vi "peg in hole Summary.vi"() -> ()   [LabVIEW 2013]
uses:
  <vilib>/Utility/file.llb/Write To Spreadsheet File (string).vi
  <vilib>/Utility/file.llb/Write To Spreadsheet File (DBL).vi
panel:
  in  "2015-03-02":dbl[](array[numeric])=[27.75, 28.05, 27.9, 17.75, 143.25, 110.6, 42.95, 17.2, 41.6, 16.8, 27.95, 65.9, 30.25, 18.5, 17.5, 48.1, 62.35, 17.55, 52.75, 322.0, 27.9, 27.45, 27.2, 18.0, 17.4, 27.95, 51.2, 17.55, 40.2, 171.4, 28.25, 27.85, 27.35, 17.85, 16.95, 39.3, 38.75, 17.35, 29.45, 17.2, 27.8, 28.15, 142.2, 63.6, 17.65, 89.651, 28.5, 17.55, 29.0, 17.15, 17.65, 28.45, 28.45, 42.9, 16.75, 38.55, 39.45, 17.8, 208.85, 49.9, 17.25, 37.75, 69.85, 29.9, 17.3, 17.5, 19.1, 80.35, 31.499, 80.55, 17.45, 17.65, 27.95, 40.65, 17.25, 70.15, 28.8, 17.4, 18.4, 17.55, 16.95, 50.4, 27.15, 52.5, 16.85, 17.6, 39.6, 17.35, 18.35, 17.75, 58.15, 71.55, 27.65, 107.75, 16.95, 28.75, 28.7, 17.5, 128.9, 59.35]
  in  "1 taught Point":dbl[](array[numeric])=[35.801, 15.05, 145.25, 25.05, 85.2, 31.05, 196.6, 25.1, 135.5, 25.45, 125.65, 25.3, 55.75, 147.2, 64.85, 25.35, 116.2, 35.45, 85.7, 45.3, 35.3, 15.9, 35.25, 15.45, 65.45, 15.35, 55.35, 14.55, 339.85, 14.65, 86.2, 15.7, 45.45, 15.449, 74.949, 26.0, 68.55, 36.45, 36.2, 26.55, 57.05, 16.65, 25.649, 58.1, 111.0, 25.9, 15.3, 129.8, 55.5, 15.3, 35.3, 15.25, 14.85, 14.55, 35.3, 15.35, 14.95, 15.25, 25.15, 14.6, 14.65, 25.6, 38.05, 15.95, 35.25, 14.75, 35.1, 15.15, 36.05, 15.1, 35.55, 14.85, 25.65, 36.9, 15.1, 14.9, 85.45, 14.5, 37.3, 14.6, 15.3, 15.35, 45.35, 15.25, 65.75, 35.85, 25.25, 15.6, 25.15, 15.35, 15.15, 36.3, 55.95, 15.5, 25.1, 14.5, 96.5, 14.8, 35.2, 14.5, 15.35, 15.65, 15.0, 15.25, 66.8, 15.4, 15.0, 15.35, 15.0, 15.35, 15.3, 15.4, 15.15, 15.35, 14.9, 15.2, 15.05, 15.4, 25.05, 14.65, 14.9, 15.45, 15.2, 15.35, 15.05, 15.45, 55.7, 15.15, 15.05, 15.5, 15.25, 15.65, 46.1, 15.6, 15.0, 15.05, 14.9, 15.4, 14.95, 15.0]
  in  "2 taught points":dbl[](array[numeric])=[126.95, 36.6, 65.75, 57.35, 75.85, 36.85, 25.5, 26.1, 45.8, 158.25, 25.35, 15.7, 127.05, 98.35, 76.5, 46.15, 85.8, 57.7, 54.95, 47.9, 35.75, 47.35, 66.2, 15.35, 116.3, 26.45, 66.45, 16.0, 55.95, 26.9, 148.35, 47.152, 140.1, 16.201, 65.8, 15.45, 45.25, 36.95, 35.7, 15.75, 57.499, 15.75, 36.25, 122.1, 68.25, 203.25, 36.0, 68.1, 75.65, 88.2, 75.45, 99.4, 55.4, 108.6, 45.65, 99.1, 35.75, 173.4, 35.6, 89.5, 45.9, 183.05, 35.6, 110.95, 35.4, 129.85, 35.6, 67.4, 36.15, 77.05, 35.35, 171.55, 25.2, 78.45, 98.95, 15.2, 25.05, 170.75, 35.65, 67.3, 77.85, 66.65, 65.85, 130.9, 25.1, 110.35, 46.051, 15.15, 66.35, 297.45, 25.15, 150.4, 88.0, 113.1, 36.5, 90.75, 25.75, 143.35, 56.5, 78.4, 47.55, 310.05, 15.052, 77.5, 27.3, 67.6, 45.3, 15.35, 67.3, 36.45, 15.2, 87.95, 25.45, 233.9, 25.45, 76.75, 66.9, 108.85, 25.25, 15.85, 66.9, 141.05, 98.6, 15.75, 14.9, 26.15, 25.2, 56.2, 45.35, 15.45, 25.35, 35.8, 87.5, 15.25, 35.35, 15.55, 15.05, 15.4, 14.95, 77.6]
  in  "central taught point":dbl[](array[numeric])=[27.75, 28.05, 27.9, 17.75, 143.25, 110.6, 42.95, 17.2, 41.6, 16.8, 27.95, 65.9, 30.25, 18.5, 17.5, 48.1, 62.35, 17.55, 52.75, 322.0, 27.9, 27.45, 27.2, 18.0, 17.4, 27.95, 51.2, 17.55, 40.2, 171.4, 28.25, 27.85, 27.35, 17.85, 16.95, 39.3, 38.75, 17.35, 29.45, 17.2, 27.8, 28.15, 142.2, 63.6, 17.65, 89.651, 28.5, 17.55, 29.0, 17.15, 17.65, 28.45, 28.45, 42.9, 16.75, 38.55, 39.45, 17.8, 208.85, 49.9, 17.25, 37.75, 69.85, 29.9, 17.3, 17.5, 19.1, 80.35, 31.499, 80.55, 17.45, 17.65, 27.95, 40.65, 17.25, 70.15, 28.8, 17.4, 18.4, 17.55, 16.95, 50.4, 27.15, 52.5, 16.85, 17.6, 39.6, 17.35, 18.35, 17.75, 58.15, 71.55, 27.65, 107.75, 16.95, 28.75, 28.7, 17.5, 128.9, 59.35]
  in  "2 taught Points & intervening joint pose":dbl[](array[numeric])=[45.5, 55.1, 25.05, 25.0, 25.152, 25.451, 25.3, 25.35, 25.1, 25.25, 14.55, 25.45, 34.85, 25.55, 14.8, 25.15, 86.1, 25.55, 15.2, 25.5, 25.2, 25.201, 15.05, 25.45, 15.0, 25.8, 15.05, 25.1, 15.1, 25.85, 14.9, 25.7, 25.05, 25.1, 46.0, 25.9, 15.3, 25.45, 25.2, 25.601, 14.9, 24.95, 15.2, 25.0, 45.95, 25.25, 385.0, 25.65, 15.3, 25.4, 15.2, 25.7, 14.8, 25.1, 46.75, 25.85, 15.35, 25.1, 15.35, 25.95, 15.6, 25.55, 15.45, 25.45, 14.9, 14.9, 15.1, 15.35, 14.8, 15.05, 56.95, 25.7, 15.0, 15.15, 14.95, 25.899, 15.0, 25.15, 15.4, 15.251, 14.95, 25.6, 15.4, 15.5, 15.15, 14.95, 15.15, 15.25, 15.3, 15.35, 15.251, 15.8, 15.0, 15.05, 15.25, 15.55, 15.55, 15.65, 15.051, 15.5, 15.0, 15.0, 15.1, 15.45, 15.1, 15.15, 15.05, 25.15, 15.15, 15.25, 15.25, 15.1, 14.9, 15.25, 14.85, 15.35, 14.95, 25.85, 15.3, 15.8, 15.2, 15.2, 14.9, 15.3, 14.85, 15.55, 15.25, 15.35, 15.25, 15.3, 14.9, 15.3, 14.85, 15.45, 14.85, 15.3, 15.1, 15.3, 15.05, 15.851]
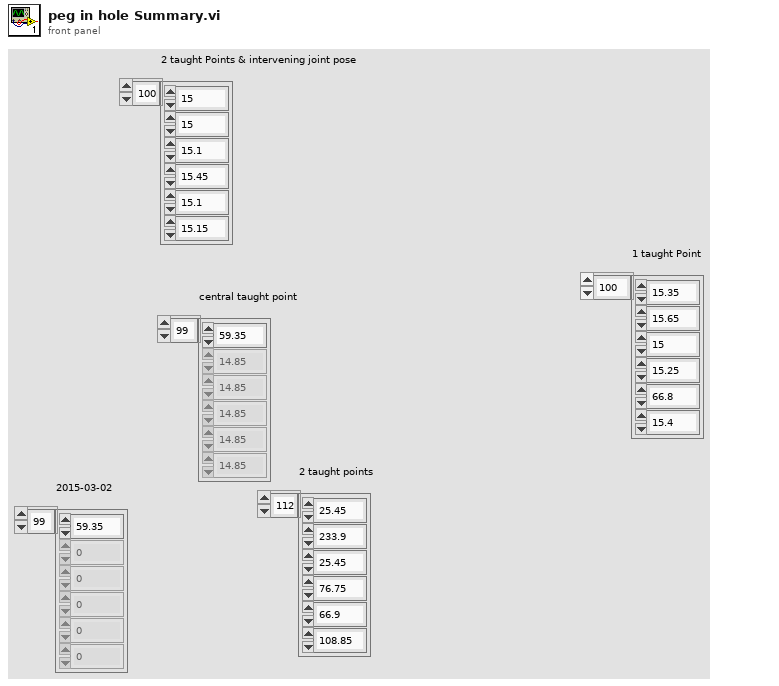
[diagram p1: front panel]
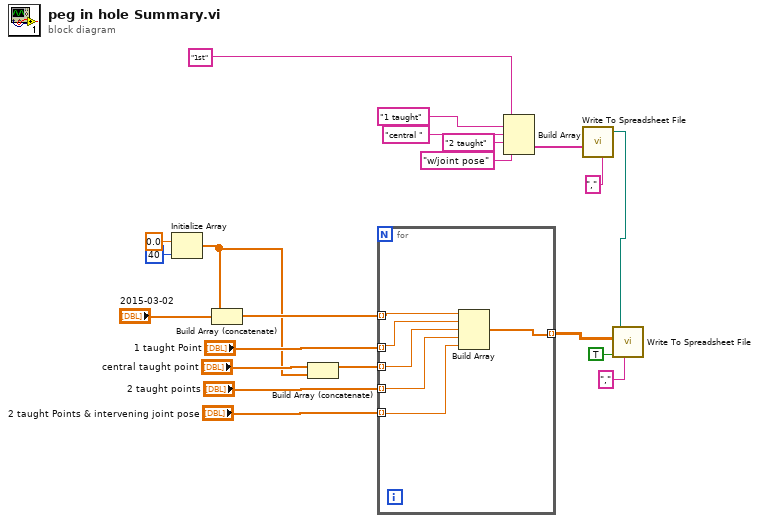
[diagram p0: block diagram]
diagram:
  n1 = Initialize Array(0.0 ("element"), 40 ("dimension size")) -> (w2:dbl[])
  n2 = Build Array (concatenate)(w2, "2015-03-02") -> (w18:dbl[])
  n3 = Build Array (concatenate)("central taught point", w2) -> (w1:dbl[])
  n4 = for {
    tunnel: w18 -> [w27] mode=indexing
    tunnel: "1 taught Point" -> [w26] mode=indexing
    tunnel: w1 -> [w25] mode=indexing
    tunnel: "2 taught points" -> [w24] mode=indexing
    tunnel: "2 taught Points & intervening joint pose" -> [w23] mode=indexing
    tunnel: [w22] -> w14 mode=indexing
    n5 = Build Array(w27, w26, w25, w24, w23) -> (w22:dbl[])
  }
  n6 = Build Array("1st", "1 taught" ("element"), "central " ("element"), "2 taught" ("element"), "w/joint pose" ("element")) -> (w6:string[])
  n7 = call-poly <vilib>:"Write To Spreadsheet File.vi"("delimiter (\\t)"="," ("delimiter (\\t)"), "1D data"=w6) -> ("new file path (Not A Path if cancelled)"=w4:path)  [unwired: 6 in]
  n8 = call-poly <vilib>:"Write To Spreadsheet File.vi"("delimiter (\\t)"="," ("delimiter (\\t)"), "append to file? (new file:F)"=TRUE, "2D data"=w14, "file path (dialog if empty)"=w4) -> ()  [unwired: 4 in, 1 out]
